vi "Integrate two peak (SubVI).vi"(0 "Time array":dbl[](array[numeric]), 1 "Start cursor index":i32, 2 "Separator cursor index":i32, 3 "End cursor index":i32, 5 "Signal array":dbl[](array[numeric]), 7 "Index cursor":dbl[](array[numeric]), 9 "Time cursor":dbl[](array[numeric]), 10 "Glu standard area":dbl format="%.6e", 11 "Signal cursor":dbl[](array[numeric]), 15 "Xyl standard area":dbl format="%.6e") -> (4 "Glu concentration":dbl format="%.4f", 6 "Xyl concentration":dbl format="%.4f", 12 "Glu area":dbl format="%.6e", 13 "Xyl area":dbl format="%.6e")   [LabVIEW 2014]
uses:
  <vilib>/Analysis/NI_AALPro.lvlib
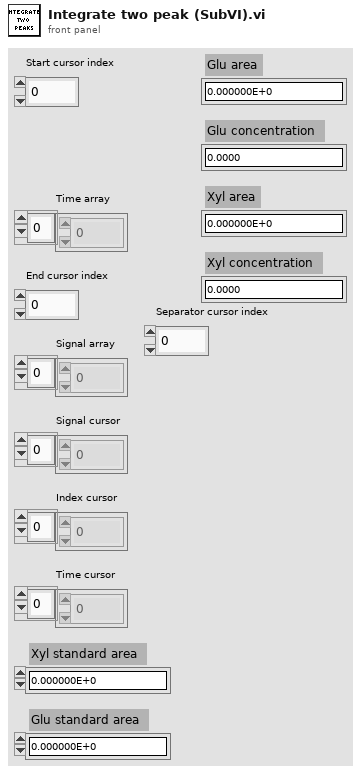
[diagram p1: front panel]
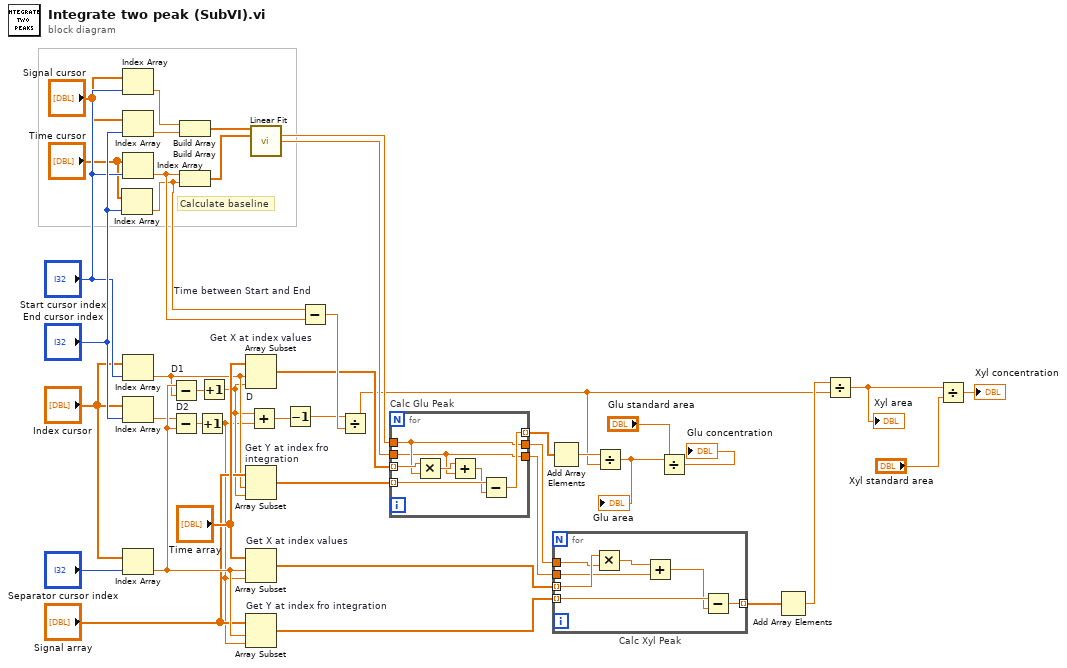
[diagram p0: block diagram]
diagram:
  # "Calculate baseline"
  n1 = Index Array(array="Time cursor", index="End cursor index") -> (element=w7:dbl)
  n2 = Index Array(array="Signal cursor", index="Start cursor index") -> (element=w19:dbl)
  n3 = Index Array(array="Signal cursor", index="End cursor index") -> (element=w20:dbl)
  n4 = Index Array(array="Time cursor", index="Start cursor index") -> (element=w8:dbl)
  n5 = Index Array(array="Index cursor", index="Start cursor index") -> (element=w9:dbl)
  n6 = Index Array(array="Index cursor", index="End cursor index") -> (element=w10:dbl)
  n7 = Index Array(array="Index cursor", index="Separator cursor index") -> (element=w35:dbl)
  n8 = Subtract "D1"(x=w35, y=w9) -> (x-y=w6:dbl)
  n9 = Subtract "D2"(x=w10, y=w35) -> (x-y=w4:dbl)
  n10 = Build Array(w19, w20) -> (w22:dbl[])
  n11 = Build Array(w8, w7) -> (w21:dbl[])
  n12 = Increment(x=w4) -> (x+1=w3:dbl)
  n13 = Increment(x=w6) -> (x+1=w5:dbl)
  n14 = Array Subset "Get X at index values"(array="Time array", index=w9, length=w5) -> (w17:dbl[])
  n15 = Array Subset "Get Y at index fro integration"(array="Signal array", index=w9, length=w5) -> (w25:dbl[])
  n16 = Array Subset "Get X at index values"(array="Time array", index=w35, length=w3) -> (w13:dbl[])
  n17 = Array Subset "Get Y at index fro integration"(array="Signal array", index=w35, length=w3) -> (w14:dbl[])
  n18 = Add "D"(x=w5, y=w3) -> (x+y=w2:dbl)
  n19 = call <vilib>:"Linear Fit.vi"("Y"=w22, "X"=w21) -> ("slope"=w24:dbl, "intercept"=w23:dbl)  [unwired: 9 in, 3 out]
  n20 = Decrement(x=w2) -> (x-1=w1:dbl)
  n21 = Subtract "Time between Start and End"(x=w7, y=w8) -> (x-y=w18:dbl)
  n22 = Divide(x=w1, y=w18) -> (x/y=w12:dbl)
  n23 = for "Calc Glu Peak" {
    tunnel: w17 -> [w50] mode=indexing
    tunnel: w25 -> [w48] mode=indexing
    tunnel: w24 -> [w45]
    tunnel: w23 -> [w44]
    tunnel: [w46] -> w33 mode=indexing
    tunnel: [w45] -> w15
    tunnel: [w44] -> w28
    n24 = Multiply(x=w50, y=w45) -> (x*y=w49:dbl)
    n25 = Add(x=w49, y=w44) -> (x+y=w47:dbl)
    n26 = Subtract(x=w48, y=w47) -> (x-y=w46:dbl)
  }
  n27 = Add Array Elements(numeric array=w33) -> (sum=w26:dbl)
  n28 = for "Calc Xyl Peak" {
    tunnel: w13 -> [w57] mode=indexing
    tunnel: w14 -> [w55] mode=indexing
    tunnel: [w53] -> w34 mode=indexing
    tunnel: w15 -> [w52]
    tunnel: w28 -> [w51]
    n29 = Multiply(x=w57, y=w52) -> (x*y=w56:dbl)
    n30 = Add(x=w56, y=w51) -> (x+y=w54:dbl)
    n31 = Subtract(x=w55, y=w54) -> (x-y=w53:dbl)
  }
  n32 = Divide(x=w26, y=w12) -> (x/y=w36:dbl)
  "Glu area" <- w36
  n33 = Divide(x=w36, y="Glu standard area") -> (x/y=→"Glu concentration":dbl)
  n34 = Add Array Elements(numeric array=w34) -> (sum=w27:dbl)
  n35 = Divide(x=w27, y=w12) -> (x/y=w39:dbl)
  "Xyl area" <- w39
  n36 = Divide(x=w39, y="Xyl standard area") -> (x/y=→"Xyl concentration":dbl)
